vi "Load Paths from Spec File.vi"(8 "error in (no error)":errorcluster, 10 "Highest Version?":bool, 11 "Spec path":path) -> (0 "error out":errorcluster, 2 "Internal Target?":bool, 3 "External Path Combinations":string[](array[string]))   [LabVIEW 2019, in "Project.Dependencies Finder.lvlib" / "Dependency Source_VIPM.lvclass"]
uses:
  Dependency Source_VIPM.lvclass
  <vilib>/Utility/config.llb/NI_LVConfig.lvlib
  Dependency Source/Dependency Source.lvclass
  Project.Dependencies Finder.lvlib
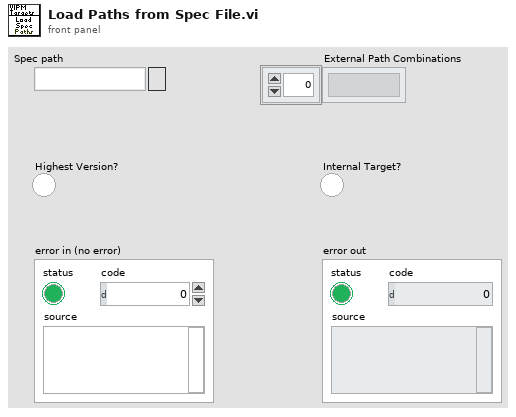
[diagram p1: front panel]
types:
  T1 = typedef "NI_LVConfig.lvlib/Config Data RefNum.ctl" = refnum<k1>
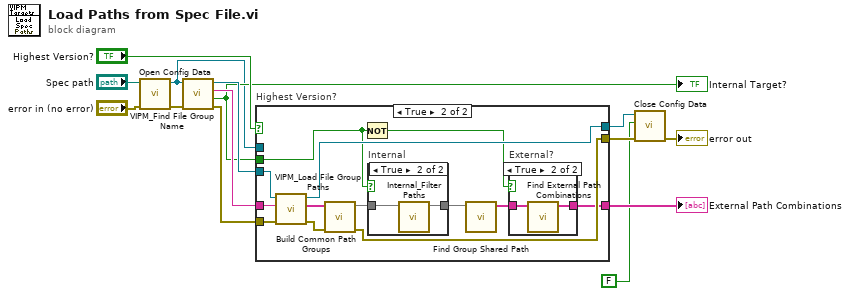
[diagram p0: block diagram]
diagram:
  n1 = call <vilib>:"Open Config Data.vi"("error in (no error)"="error in (no error)", "configuration file path"="Spec path") -> ("error out"=w2:errorcluster, "refnum"=w1:T1)  [unwired: 7 in, 1 out]
  n2 = call "VIPM_Find File Group Name.vi"("error in (no error)"=w2, "Refnum in"=w1) -> ("error out"=w9:errorcluster, "Internal Target?"=w10:bool, "File Group Name"=w11:string, "Refnum out"=w12:T1)  [unwired: 6 in]
  "Internal Target?" <- w10
  n3 = case "Highest Version?" shown="True" "Highest Version?" {
    tunnel: w1 -> [w16 _]
    tunnel: [w16 w29] -> w3
    tunnel: [w15 w26] -> w5
    tunnel: [_ w21] -> w6
    tunnel: w9 -> [w15 w20]
    tunnel: w10 -> [_ w19]
    tunnel: w11 -> [_ w18]
    tunnel: w12 -> [_ w17]
    frame False {
    }
    frame True {
      n4 = call "VIPM_Load File Group Paths.vi"("error in (no error)"=w20, "File Group Name"=w18, "Refnum in"=w17) -> ("error out"=w28:errorcluster, "File Group Paths"=w27:string[], "Refnum out"=w29:T1)  [unwired: 6 in]
      n5 = call "Build Common Path Groups.vi"("error in (no error)"=w28, "File Group Paths"=w27) -> ("error out"=w26:errorcluster, "Common Path map"=w25:map{string, string[]})  [unwired: 8 in]
      n6 = Not(x=w19) -> (.not. x?=w23:bool)
      n7 = case "Internal" shown="True" w19 {
        tunnel: w25 -> [w33 w35]
        tunnel: [w33 w34] -> w24
        frame False {
        }
        frame True {
          n8 = call "Internal_Filter Paths.vi"("Unfiltered path map in"=w35) -> ("Filtered path map out"=w34:map{string, string[]})  [unwired: 10 in]
        }
      }
      n9 = call "Find Group Shared Path.vi"("Group Filtered Path map"=w24) -> ("Found Common Paths"=w22:string[])  [unwired: 10 in]
      n10 = case "External?" shown="True" w23 {
        tunnel: [w30 w31] -> w21
        tunnel: w22 -> [w30 w32]
        frame False {
        }
        frame True {
          n11 = call "Find External Path Combinations.vi"("Found Common Paths in"=w32) -> ("External Path Combinations"=w31:string[])  [unwired: 10 in]
        }
      }
    }
  }
  "External Path Combinations" <- w6
  n12 = call <vilib>:"Close Config Data.vi"("error in (no error)"=w5, "write file if changed (T)"=FALSE, "refnum"=w3) -> ("error out"=→"error out":errorcluster)  [unwired: 7 in, 1 out]
